vi "Row_Set Cell Values (text).vi"(8 "error in (no error)":errorcluster, 9 "text data (row)":string[](array[string]), 10 "Row":refnum<k24>, 11 "ooWriter in":refnum<class "ooWriter.lvclass">) -> (0 "error out":errorcluster, 3 "ooWriter out":refnum<class "ooWriter.lvclass">)   [LabVIEW 2009, in "ooWriter.lvclass"]
uses:
  ooWriter.lvclass
  C:/Projets/LAVAG/OpenOfficeRGT/AODL/DLLs/AODL.dll
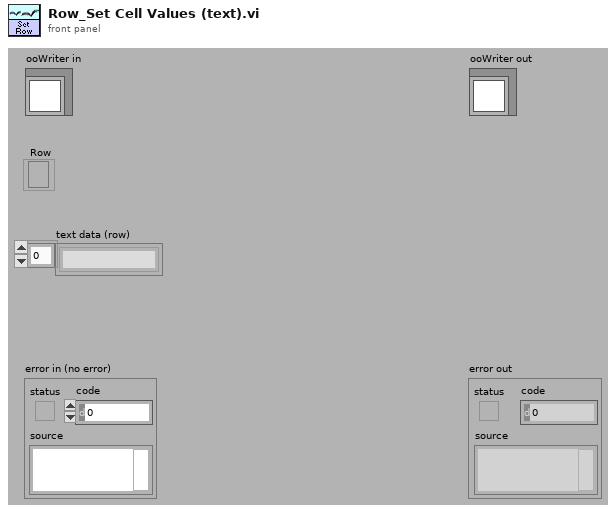
[diagram p1: front panel]
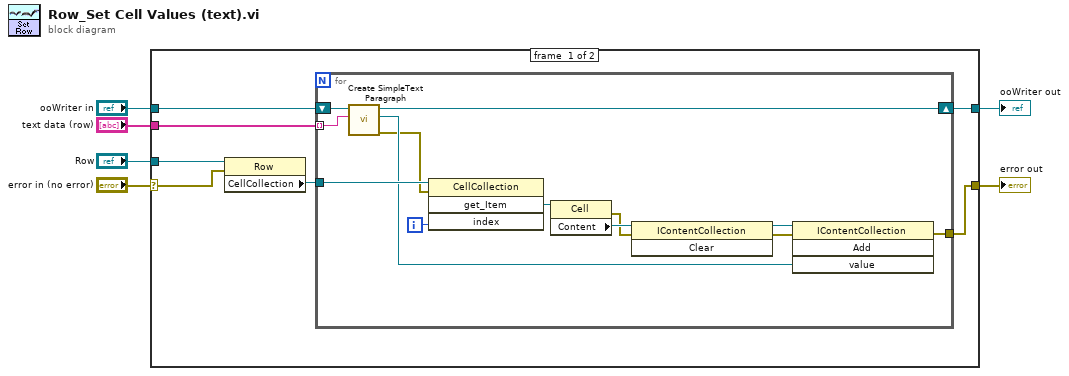
[diagram p0: block diagram]
diagram:
  n1 = case shown="No Error" "error in (no error)" {
    selector: "error in (no error)" -> [w10 w28]
    tunnel: [w9 w28] -> w5
    tunnel: [w7 w27] -> w3
    tunnel: "ooWriter in" -> [w8 w27]
    tunnel: "text data (row)" -> [w12 _]
    tunnel: "Row" -> [w11 _]
    frame #0 {
      n2 = property class="Row"(reference=w11, error in=w10) -> ("CellCollection"=w13:refnum<k24>)  [unwired: 2 out]
      n3 = for {
        tunnel: [w25] -> w9
        tunnel: w13 -> [w24]
        tunnel: w12 -> [w21] mode=indexing
        shift-right: [w19] -> w7
        shift-left: w8 -> [w22]
        i -> [w23]
        n4 = call-dynamic "Create SimpleText Paragraph.vi"("simpleText"=w21, "ooWriter in"=w22) -> ("error out"=w18:errorcluster, "SimpleTextParagraph"=w20:refnum<k24>, "ooWriter out"=w19:refnum<class "ooWriter.lvclass">)  [unwired: 7 in]
        n5 = invoke class="CellCollection" method="get_Item"(reference=w24, error in=w18, "index"=w23) -> ("get_Item"=w26:refnum<k24>)  [unwired: 1 in, 3 out]
        n6 = property class="Cell"(reference=w26) -> (error out=w15:errorcluster, "Content"=w17:refnum<k24>)  [unwired: 1 in, 1 out]
        n7 = invoke class="IContentCollection" method="Clear"(reference=w17, error in=w15) -> (reference out=w16:refnum<k24>, error out=w14:errorcluster)  [unwired: 1 in, 1 out]
        n8 = invoke class="IContentCollection" method="Add"(reference=w16, error in=w14, "value"=w20) -> (error out=w25:errorcluster)  [unwired: 1 in, 3 out]
      }
    }
    frame #1 {
    }
  }
  "error out" <- w5
  "ooWriter out" <- w3
